vi "Get Scanner.vi"(8 "error in (no error)":errorcluster, 11 "Varian Magnet in":refnum<class "Varian Magnet.lvclass">) -> (0 "error out":errorcluster, 2 "Default Scanner out":refnum<class "Scanner.lvclass">)   [LabVIEW 2009, in "Varian Magnet.lvclass"]
doc: "(Dynamic) Returns the default Scanner object that scans over this Scannable. (Note that a Scannable may have multiple Scanners associated with it.) A Scanner is an analogue to an Iterator class in other languages."
uses:
  Varian Magnet.lvclass
  Scanners/Scanner/Scanner.lvclass
  Utility Classes/Scannable/Scannable.lvclass
  Scans/Varian Magnet Scan/Varian Magnet Scan.lvclass
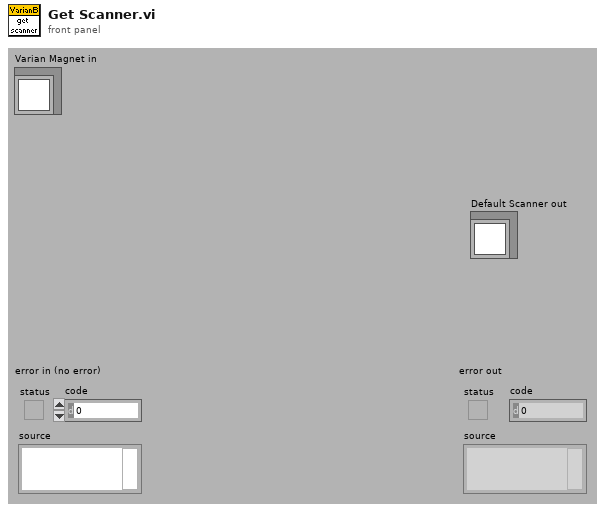
[diagram p1: front panel]
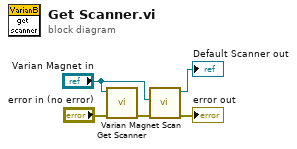
[diagram p0: block diagram]
diagram:
  n1 = call-parent "Get Scanner.vi"("error in (no error)"="error in (no error)", "Scannable in"="Varian Magnet in") -> ("error out"=w2:errorcluster)  [unwired: 9 out]
  n2 = call "Varian Magnet Scan.vi"("error in (no error)"=w2, "Varian Magnet.lvclass"="Varian Magnet in") -> ("error out"=→"error out":errorcluster, "Varian Magnet Scan out"=→"Default Scanner out":refnum<class "Varian Magnet Scan.lvclass">)  [unwired: 8 out]
